vi "TestStringSinkNoBufferAllEventsCaptured.vi"(8 "error in (no error)":errorcluster, 11 "TestCase in":refnum<class "TestStringControlSink.lvclass">) -> (0 "error out":errorcluster, 3 "TestCase out":refnum<class "TestStringControlSink.lvclass">)   [LabVIEW 2019, in "TestStringControlSink.lvclass"]
uses:
  TestStringControlSink.lvclass
  Source/String Formats/String Expression Format/String Expression Format.lvclass/String Expression Format.ctl
  Source/Composed Log/LoggerReference/LoggerReference.lvclass/LoggerReference.ctl
  7fc97478-71b4-4be4-9b40-44a1edbd2178.vi
  1ec4c22a-6b03-4cff-a1e2-0f91a771adcd.vi
  Source/String Formats/String Expression Format/Run Formatter.vi
  Source/Composed Log/LoggerReference/Return Aggregate Queues.vi
  Source/Composed Log/LoggerReference/Add Aggregate Log.vi
  7fc97478-71b4-4be4-9b40-44a1edbd2178.vi/af3b3336-f291-42a8-9b57-711866ed8ead.vi
  Source/Composed Log/LoggerReference/Log.vi
  Source/Composed Log/LoggerReference/Get Valid Event Time.vi
  <vilib>/dlg_ctls.llb/Space Constant.vi
  Source/Composed Log/LoggerReference/Send Add Sink.vi
  Source/Composed Log/LoggerReference/Remove Stale Logs.vi
  Source/String Formats/String Expression Format/String Expression Format.lvclass
  C:/CS/Log/Source/IStringFormat/IStringFormat.lvclass
  Source/String Control Sink/String Control Sink.lvclass
  C:/CS/Log/Source/Composed Log/Log Sink/Log Sink.lvclass
  Source/Composed Log/Application Logger/Launch Worker Loop.vi
  Source/Composed Log/LoggerReference/Initialize Logger Instance.vi
  Source/Composed Log/LoggerReference/LoggerReference.lvclass
  Source/Composed Log/IErrorFormat/IErrorFormat.lvclass
  Source/Composed Log/Log Sink/Log Sink.lvclass
  <vilib>/addons/_JKI Toolkits/VI Tester/TestCase.llb/TestCase.lvclass
  C:/Program Files (x86)/National Instruments/LabVIEW 2019/vi.lib/addons/_JKI Toolkits/VI Tester/TestCase.llb/TestCase.lvclass
panel:
  out "String":string
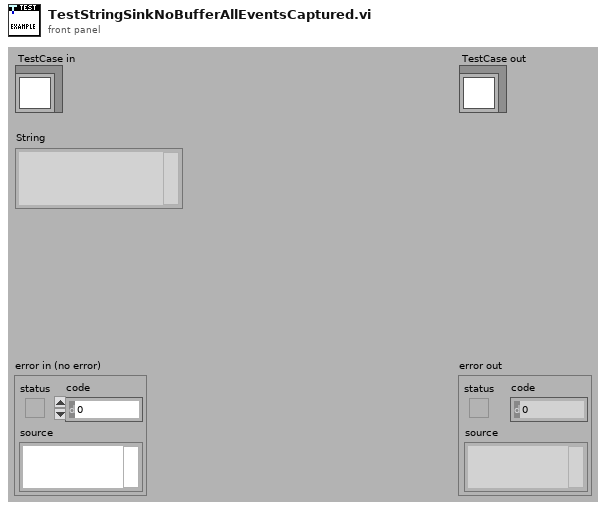
[diagram p1: front panel]
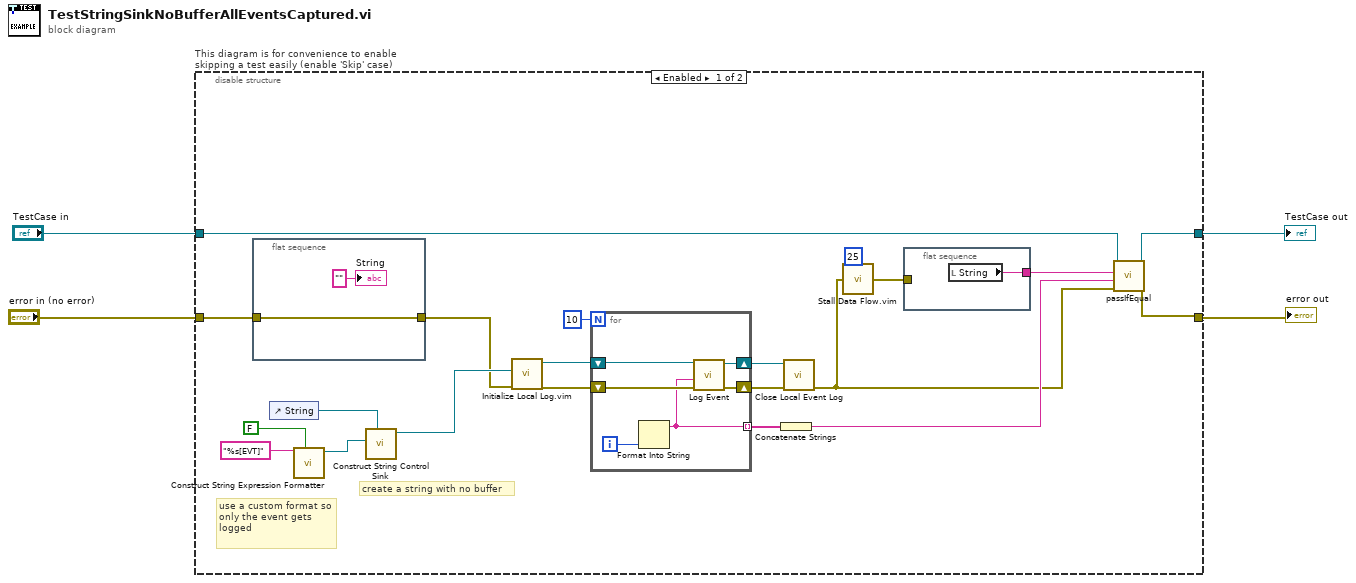
[diagram p0: block diagram]
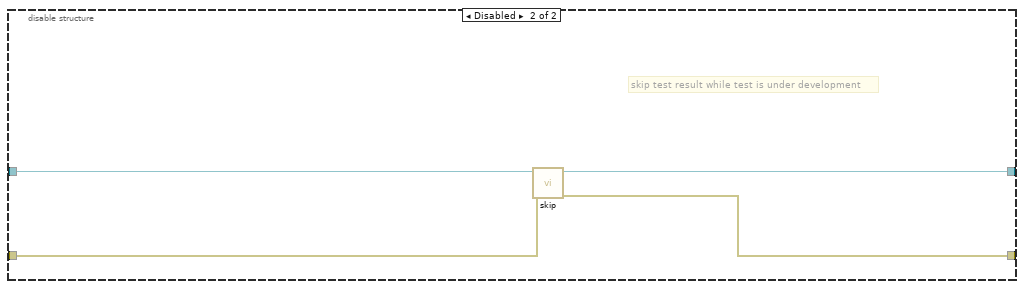
[diagram p2: hidden frame]
diagram:
  n1 = disable-structure "This diagram is for convenience to enable skipping a test easily (enable 'Skip' case)" shown="Enabled" {
    disable-tunnel: "TestCase in" -> [w25 w38]
    disable-tunnel: [w24 w36] -> w1
    disable-tunnel: [w23 w37] -> w3
    disable-tunnel: "error in (no error)" -> [w6 w35]
    frame Enabled {
      # "create a string with no buffer"
      # "use a custom format so only the event gets logged"
      n2 = flat-sequence {
        tunnel: w6 -> [w27]
        tunnel: [w27] -> w5
        frame #0 {
          "String" <- "" ("String")
        }
      }
      n3 = control-ref of="String"() -> (w22:refnum<vi>)
      n4 = call "Construct String Expression Formatter.vi"("Append EOL?"=FALSE, "Format Specifier"="%s[EVT]") -> ("String Expression Format out"=w20:refnum<class "String Expression Format.lvclass">)  [unwired: 8 in, 1 out]
      n5 = call "Construct String Control Sink.vi"("Str Refnum"=w22, "LogFormat"=w20) -> ("String Control Sink out"=w19:refnum<class "String Control Sink.lvclass">)  [unwired: 9 in]
      n6 = call "Initialize Local Log.vim"("error in (no error)"=w5, "Startup Sink(s)"=w19) -> ("error out"=w17:errorcluster, "Log Instance Reference"=w18:refnum<class "LoggerReference.lvclass">)  [unwired: 7 in, 1 out]
      n7 = for {
        N: 10 -> [_]
        shift-right: [w32] -> w14
        shift-left: w17 -> [w33]
        tunnel: [w30] -> w12 mode=indexing
        shift-right: [w29] -> w13
        shift-left: w18 -> [w34]
        i -> [w31]
        n8 = Format Into String(w31) -> (resulting string=w30:string)  [unwired: 3 in, 1 out]
        n9 = call "Log Event.vi"("error in (no error)"=w33, "Data To Log"=w30, "Log Instance"=w34) -> ("error out"=w32:errorcluster, "Log Instance Out"=w29:refnum<class "LoggerReference.lvclass">)  [unwired: 7 in]
      }
      n10 = Concatenate Strings(w12) -> (w11:string)
      n11 = call "Close Local Event Log.vi"("error in (no error)"=w14, "Log Instance"=w13) -> ("error out"=w9:errorcluster)  [unwired: 9 in]
      n12 = call "Stall Data Flow.vim"("value in"=w9, "milliseconds to wait"=u32 25) -> ("value out"=w8:errorcluster)  [unwired: 1 out]
      n13 = flat-sequence {
        tunnel: [w28] -> w10
        tunnel: w8 -> [_]
        frame #0 {
          n14 = local read "String"() -> (w28:string)
        }
      }
      n15 = call-dynamic "passIfEqual.vi"("error in (no error)"=w9, "y"=w11, "x"=w10, "TestCase in"=w25) -> ("error out"=w23:errorcluster, "TestCase out"=w24:refnum<class "TestStringControlSink.lvclass">)  [unwired: 6 in]
    }
    frame Disabled {
      # "skip test result while test is under development"
      n16 = call <vilib>:"skip.vi"("error in (no error)"=w35, "TestCase in"=w38) -> ("error out"=w37:errorcluster, "TestCase out"=w36:refnum<class "TestStringControlSink.lvclass">)  [unwired: 8 in]
    }
  }
  "error out" <- w3
  "TestCase out" <- w1
